vi "ArrayControls.vi"() -> ()   [LabVIEW 2016, in "test_ValueSignal.lvlib"]
uses:
  test_ValueSignal.lvlib
  Helper/HelperVI1-array.vi
  main/apis/Stimulus/ValueSignalByPathString.vi
  main/apis/Assert/AssertControlValueByPathString.vi
  <vilib>/addons/_JKI Toolkits/Caraya/classes/Assert/Assert Equal Value_Variant.vi
  <vilib>/addons/_JKI Toolkits/Caraya/classes/Assert/Assert.lvclass
  <vilib>/addons/_JKI Toolkits/Caraya/classes/Test/Test.lvclass
panel:
  out "error out":errorcluster
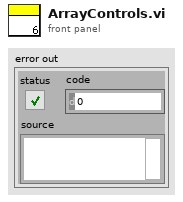
[diagram p1: front panel]
types:
  T1 = cluster{"Numeric":dbl, "String":string, "Boolean":bool}[]
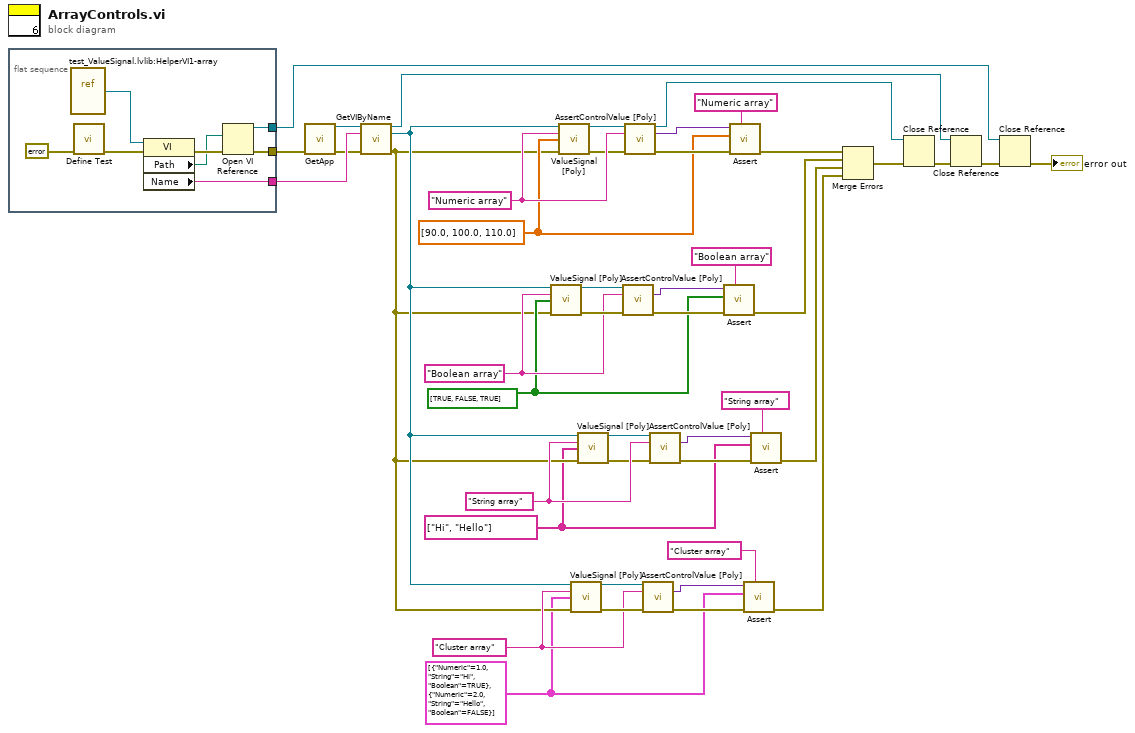
[diagram p0: block diagram]
diagram:
  w2 = T1 [{"Numeric"=1.0, "String"="Hi", "Boolean"=TRUE}, {"Numeric"=2.0, "String"="Hello", "Boolean"=FALSE}] ("Cluster array")
  w8 = "Cluster array" ("Class Name")
  w1 = string[] ["Hi", "Hello"]
  w16 = "String array" ("Class Name")
  w19 = bool[] [TRUE, FALSE, TRUE]
  w24 = "Boolean array" ("Class Name")
  w21 = dbl[] [90.0, 100.0, 110.0]
  w36 = "Numeric array" ("Class Name")
  n1 = flat-sequence {
    tunnel: [w49] -> w40
    tunnel: [w48] -> w42
    tunnel: [w46] -> w39
    frame #0 {
      n2 = vi-ref "test_ValueSignal.lvlib:HelperVI1-array.vi"() -> (w51:refnum<vi>)
      n3 = call <vilib>:"Define Test.vi"("error in (no error)"=errorcluster {"status"=FALSE, "code"=0, "source"=""}) -> ("error out"=w52:errorcluster)  [unwired: 10 in]
      n4 = property on="Property Node" class="VI"(reference=w51, error in=w52) -> (error out=w50:errorcluster, "Path"=w47:path, "Name"=w46:string)  [unwired: 1 out]
      n5 = Open VI Reference(vi path=w47, error in (no error)=w50) -> (vi reference=w48:refnum<vi>, error out=w49:errorcluster)  [unwired: 4 in]
    }
  }
  n6 = call "GetApp.vi"("error in (no error)"=w40) -> ("Application Ref"=w41:refnum<vi>, "error out"=w38:errorcluster)  [unwired: 13 in]
  n7 = call "GetVIByName.vi"("Application Ref in"=w41, "VI Name"=w39, "error in (no error)"=w38) -> ("Application Ref out"=w28:refnum<vi>, "VI Reference"=w5:refnum<vi>, "error out"=w4:errorcluster)  [unwired: 10 in]
  n8 = call-poly "ValueSignal [Poly].vi"("VI Reference In"=w5, "Control Name"=w24, "Value (Signaling)"=w19, "error in"=w4) -> ("VI Reference Out"=w23:refnum<vi>, "error out"=w25:errorcluster)  [unwired: 10 in]
  n9 = call-poly "ValueSignal [Poly].vi"("VI Reference In"=w5, "Control Name"=w36, "Value (Signaling)"=w21, "error in"=w4) -> ("VI Reference Out"=w37:refnum<vi>, "error out"=w35:errorcluster)  [unwired: 10 in]
  n10 = call-poly "ValueSignal [Poly].vi"("VI Reference In"=w5, "Control Name"=w8, "Value (Signaling)"=w2, "error in"=w4) -> ("VI Reference Out"=w7:refnum<vi>, "error out"=w9:errorcluster)  [unwired: 10 in]
  n11 = call-poly "ValueSignal [Poly].vi"("VI Reference In"=w5, "Control Name"=w16, "Value (Signaling)"=w1, "error in"=w4) -> ("VI Reference Out"=w17:refnum<vi>, "error out"=w15:errorcluster)  [unwired: 10 in]
  n12 = call-poly "AssertControlValue [Poly].vi"("VI Reference In"=w23, "Control Name"=w24, "error in"=w25) -> ("Value"=w27:variant, "error out"=w26:errorcluster)  [unwired: 10 in, 1 out]
  n13 = call-poly "AssertControlValue [Poly].vi"("VI Reference In"=w37, "Control Name"=w36, "error in"=w35) -> ("VI Reference Out"=w30:refnum<vi>, "Value"=w33:variant, "error out"=w34:errorcluster)  [unwired: 10 in]
  n14 = call-poly "AssertControlValue [Poly].vi"("VI Reference In"=w7, "Control Name"=w8, "error in"=w9) -> ("Value"=w11:variant, "error out"=w10:errorcluster)  [unwired: 10 in, 1 out]
  n15 = call-poly "AssertControlValue [Poly].vi"("VI Reference In"=w17, "Control Name"=w16, "error in"=w15) -> ("Value"=w13:variant, "error out"=w14:errorcluster)  [unwired: 10 in, 1 out]
  n16 = call-poly <vilib>:"Assert.vi"("Label"="Boolean array" ("Label (VI Title)"), "error in (no error)"=w26, "Y"=w19, "X"=w27) -> ("error out"=w20:errorcluster)  [unwired: 7 in]
  n17 = call-poly <vilib>:"Assert.vi"("Label"="Numeric array" ("Label (VI Title)"), "error in (no error)"=w34, "Y"=w21, "X"=w33) -> ("error out"=w44:errorcluster)  [unwired: 7 in]
  n18 = call-poly <vilib>:"Assert.vi"("Label"="Cluster array" ("Label (VI Title)"), "error in (no error)"=w10, "Y"=w2, "X"=w11) -> ("error out"=w3:errorcluster)  [unwired: 7 in]
  n19 = call-poly <vilib>:"Assert.vi"("Label"="String array" ("Label (VI Title)"), "error in (no error)"=w14, "Y"=w1, "X"=w13) -> ("error out"=w12:errorcluster)  [unwired: 7 in]
  n20 = Merge Errors(w44, w20, w12, w3) -> (w32:errorcluster)
  n21 = Close Reference(reference=w30, error in (no error)=w32) -> (error out=w31:errorcluster)
  n22 = Close Reference(reference=w28, error in (no error)=w31) -> (error out=w29:errorcluster)
  n23 = Close Reference(reference=w42, error in (no error)=w29) -> (error out=→"error out":errorcluster)
